vi "接收百分比.vi"(8 "需发送次数":i32, 9 "帧数":i32, 10 "帧号":i32, 11 "已收次数":i32) -> (1 "已收百分比":string, 2 "已收百分比":u8)   [LabVIEW 2016, in "数据传输系统-02.lvlib" / "自动更新.lvlib" / "TCP文件传输系统.lvlib" / "TCP接收文件.lvlib"]
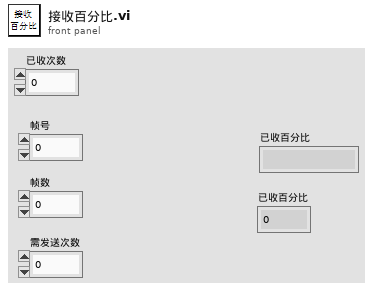
[diagram p1: front panel]
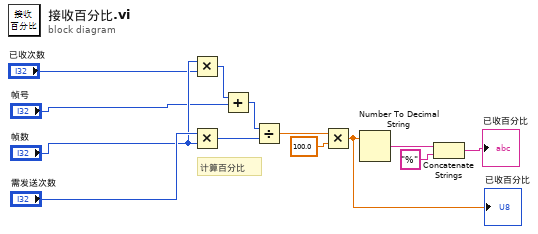
[diagram p0: block diagram]
diagram:
  # "计算百分比"
  n1 = Multiply(x="帧数", y="已收次数") -> (x*y=w5:i32)
  n2 = Multiply(x="需发送次数", y="帧数") -> (x*y=w7:i32)
  n3 = Add(x=w5, y="帧号") -> (x+y=w6:i32)
  n4 = Divide(x=w6, y=w7) -> (x/y=w8:dbl)
  n5 = Multiply(x=w8, y=100.0) -> (x*y=w10:dbl)
  "已收百分比" <- w10
  n6 = Number To Decimal String(number=w10) -> (decimal integer string=w11:string)  [unwired: 1 in]
  n7 = Concatenate Strings(w11, "%" ("字符串")) -> (→"已收百分比":string)
